vi "roboRIO v1.0 Configure SPI.vi"(8 "error in (no error)":errorcluster, 9 "SPI Configuration v1.0":T4 {"Frame Length" min=1 max=16}, 10 "SPI Channel":T1, 11 "myRIO Ref In":T2) -> (0 "error out":errorcluster, 3 "Actual Frequency (Hz)":dbl)   [LabVIEW 2021]
uses:
  <vilib>/myRIO/Common/Instrument Driver Framework/myRIO v1.0/SPI/typedefs/SPI Configuration v1.0.ctl
  <vilib>/myRIO/Common/Instrument Driver Framework/myRIO v1.0/SPI/typedefs/SPI Clock Phase.ctl
  <vilib>/myRIO/Common/Instrument Driver Framework/myRIO v1.0/SPI/typedefs/SPI Clock Polarity.ctl
  <vilib>/myRIO/Common/Instrument Driver Framework/myRIO v1.0/SPI/typedefs/SPI Data Direction.ctl
  <vilib>/myRIO/Common/Instrument Driver Framework/myRIO v1.0/SPI/typedefs/SPI Frame Length.ctl
  <vilib>/myRIO/Common/Instrument Driver Framework/Utilities/typedefs/myRIO v1.0 Reference.ctl
  <vilib>/myRIO/Common/Instrument Driver Framework/Utilities/typedefs/Generic FPGA Reference.ctl
  <vilib>/myRIO/Common/Instrument Driver Framework/myRIO v1.0/SPI/typedefs/SPI Channels Enum.ctl
  <vilib>/myRIO/Common/Instrument Driver Framework/roboRIO v1.0/SPI/typedefs/roboRIO SPI Channels FPGA Reference.ctl
  <vilib>/myRIO/Common/Instrument Driver Framework/Utilities/vis/Calculate Clock Settings.vi
  <vilib>/myRIO/Common/Instrument Driver Framework/Utilities/vis/Calculate TOP (Phase Correct Mode).vi
  <vilib>/myRIO/Common/Instrument Driver Framework/Utilities/vis/Calculate TOP (Normal Mode).vi
  <vilib>/myRIO/Common/Instrument Driver Framework/Utilities/vis/Calculate Frequency (Phase Correct Mode).vi
  <vilib>/myRIO/Common/Instrument Driver Framework/Utilities/vis/Calculate Frequency (Normal Mode).vi
  <vilib>/rvi/errors/niLvFpgaAdjustHostInterfaceError.vi
  <vilib>/rvi/interface/nirviReadWriteControl/nirviReadWriteControl.xnode
  <vilib>/rvi/interface/Simulation/niFpgaSimulationCallBeginRW.vi
  NiFpgaLv.dll
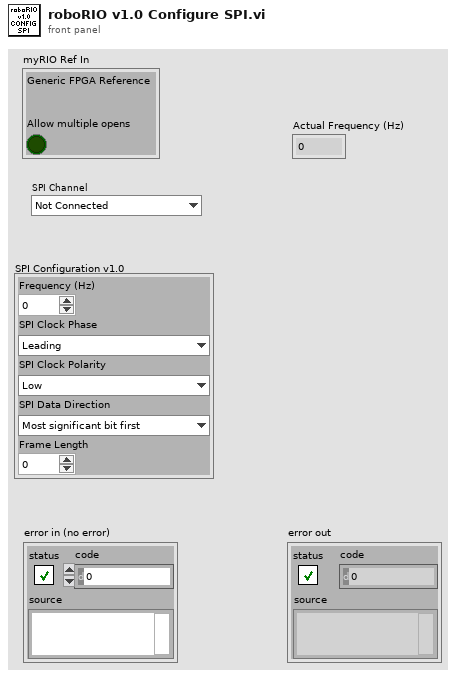
[diagram p1: front panel]
types:
  T1 = typedef "SPI Channels Enum.ctl" = enum16{"Not Connected", "A/SPI", "B/SPI", "SPI/SPI"}
  T2 = typedef "myRIO v1.0 Reference.ctl" = cluster{"Generic FPGA Reference":T3, "Allow multiple opens":bool}
  T3 = typedef "Generic FPGA Reference.ctl" = refnum<k20>
  T4 = typedef "SPI Configuration v1.0.ctl" = cluster{"Frequency (Hz)":dbl, "SPI Clock Phase":T5, "SPI Clock Polarity":T6, "SPI Data Direction":T7, "Frame Length":T8}
  T5 = typedef "SPI Clock Phase.ctl" = enum8{"Leading", "Trailing"}
  T6 = typedef "SPI Clock Polarity.ctl" = enum8{"Low", "High"}
  T7 = typedef "SPI Data Direction.ctl" = enum8{"Most significant bit first", "Least significant bit first"}
  T8 = typedef "SPI Frame Length.ctl" = u8
  T9 = typedef "roboRIO SPI Channels FPGA Reference.ctl" = refnum<k20>
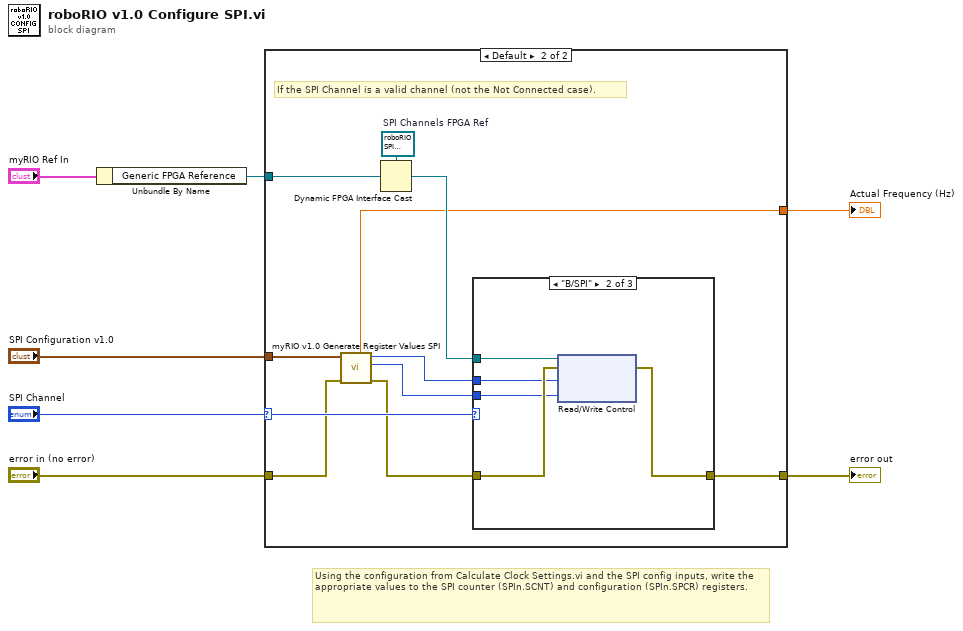
[diagram p0: block diagram]
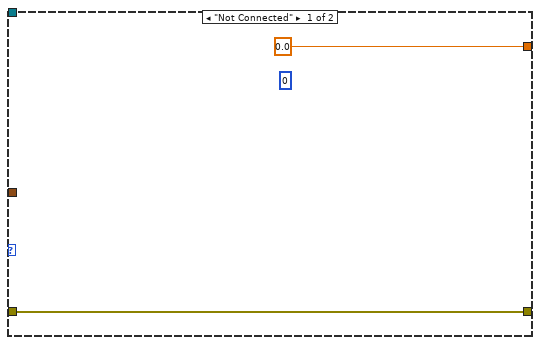
[diagram p2: hidden frame]
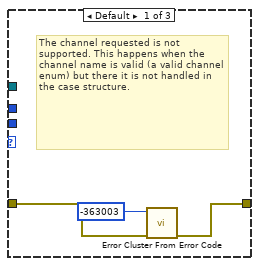
[diagram p3: hidden frame]
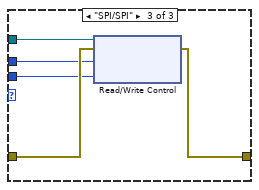
[diagram p4: hidden frame]
diagram:
  # "Using the configuration from Calculate Clock Settings.vi and the SPI config inputs, write the appropriate values to the SPI counter (SPIn.SCNT) and configuration (SPIn.SPCR) registers."
  n1 = Unbundle By Name("myRIO Ref In") -> ("Generic FPGA Reference"=w1:T3)
  n2 = case shown="Default" "SPI Channel" {
    selector: "SPI Channel" -> [_ w16]
    tunnel: [w8 w18] -> w7
    tunnel: "SPI Configuration v1.0" -> [_ w10]
    tunnel: "error in (no error)" -> [w8 w15]
    tunnel: w1 -> [_ w17]
    tunnel: [0.0 ("Actual Frequency (Hz)") w11] -> w2
    frame "Not Connected" {
      (unwired) u16 0
    }
    frame Default {
      w20 = T9 refnum  # SPI Channels FPGA Ref
      # "If the SPI Channel is a valid channel (not the Not Connected case)."
      n3 = call <vilib>:"myRIO v1.0 Generate Register Values SPI.vi"("error in (no error)"=w15, "SPI Configuration v1.0"=w10) -> ("error out"=w14:errorcluster, "SPI.CNFG"=w12:u16, "SPI.CNT"=w13:u16, "Actual Frequency (Hz)"=w11:dbl)  [unwired: 6 in]
      n4 = Dynamic FPGA Interface Cast(Session In=w20, Type=w17) -> (Session Out=w19:T9)
      n5 = case shown="\"B/SPI\"" w16 {
        tunnel: w14 -> [w21 w28 w33]
        tunnel: [w22 w27 w32] -> w18
        tunnel: w19 -> [_ w26 w31]
        tunnel: w13 -> [_ w25 w30]
        tunnel: w12 -> [_ w24 w29]
        frame Default {
          # "The channel requested is not supported. This happens when the channel name is valid (a valid channel enum) but there it is not handled in the case structure."
          n6 = call <vilib>:"Error Cluster From Error Code.vi"("error in (no error)"=w21, "error code (0)"=-363003) -> ("error out"=w22:errorcluster)  [unwired: 7 in]
        }
        frame "B/SPI" {
          n7 = xnode "Read/Write Control"("FPGA VI Reference In"=w26, "error in"=w28, "SPI.B.CNT"=w25, "SPI.B.CNFG"=w24) -> ("error out"=w27:errorcluster)  [unwired: 1 out]
        }
        frame "SPI/SPI" {
          n8 = xnode "Read/Write Control"("FPGA VI Reference In"=w31, "error in"=w33, "SPI.SPI.CNT"=w30, "SPI.SPI.CNFG"=w29) -> ("error out"=w32:errorcluster)  [unwired: 1 out]
        }
      }
    }
  }
  "error out" <- w7
  "Actual Frequency (Hz)" <- w2
